vi "Set RFPM Private Boolean Attribute Value.vi"(0 "reference":refnum<k15>, 5 "Attribute":i32(ring)=10 items=["Source Cal Correct Mismatch"=10, "Perform Limited System Cal?"=20], 7 "value":bool, 11 "error in":errorcluster {"code" format="%.0x"}) -> (4 "reference out":refnum<k15>, 15 "error out":errorcluster {"code" format="%.0x"})   [LabVIEW 2023, in "RFFixtureCharact.RFPM.lvlib" / "RF Subsystem Session Provider.lvclass"]
uses:
  RF Subsystem Session Provider.lvclass
  ivi.dll
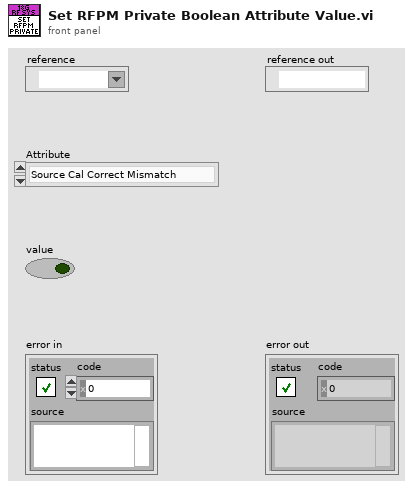
[diagram p1: front panel]
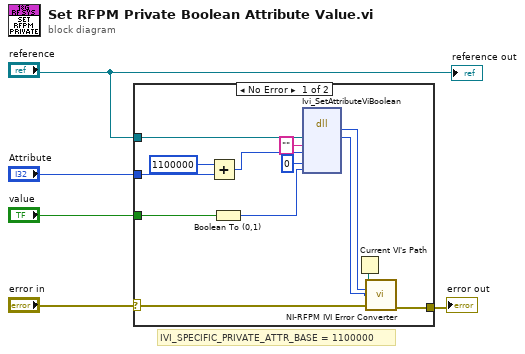
[diagram p0: block diagram]
diagram:
  # "IVI_SPECIFIC_PRIVATE_ATTR_BASE = 1100000"
  n1 = case shown="No Error" "error in" {
    selector: "error in" -> [w6 w19]
    tunnel: [w17 w19] -> w5
    tunnel: "reference" -> [w18 _]
    tunnel: "Attribute" -> [w10 _]
    tunnel: "value" -> [w7 _]
    frame No Error {
      n2 = Add(x=1100000, y=w10) -> (x+y=w12:i32)
      n3 = Boolean To (0,1)(Boolean=w7) -> (0, 1=w8:i16)
      n4 = dll-call lib="ivi.dll" fn="Ivi_SetAttributeViBoolean" ("ni5530CalUtility.dll:ni5530CalUtility_InitiateCalibration")("Session"=w18, "channel"="", "attribID"=w12, "flags"=0, "value"=w8) -> ("return type"=w15:i32, "Session"=w16:u32)  [unwired: 3 in, 6 out]
      n5 = Current VI's Path() -> (path=w14:path)
      n6 = call <instrlib>:"NI-RFPM IVI Error Converter.vi"("path to vi"=w14, "ivi error code"=w15, "instrument handle"=w16, "error in"=w6) -> ("error out"=w17:errorcluster)  [unwired: 11 in]
    }
    frame Error {
    }
  }
  "error out" <- w5
  "reference out" <- "reference"
